vi "CMD_RETURN.vi"(6 "Gantry in":refnum<class "Gantry.lvclass">, 8 "error in (no error)":errorcluster, 10 "Arguments":string[](array[string]), 11 "gScript Interpreter in":refnum<class "gScript Interpreter.lvclass">) -> (0 "error out":errorcluster, 3 "gScript Interpreter out":refnum<class "gScript Interpreter.lvclass">, 4 "Gantry out":refnum<class "Gantry.lvclass">)   [LabVIEW 2024, in "gScript Interpreter.lvclass"]
uses:
  gScript Interpreter.lvclass
  Shared Components/Gantry Class/Gantry.lvclass
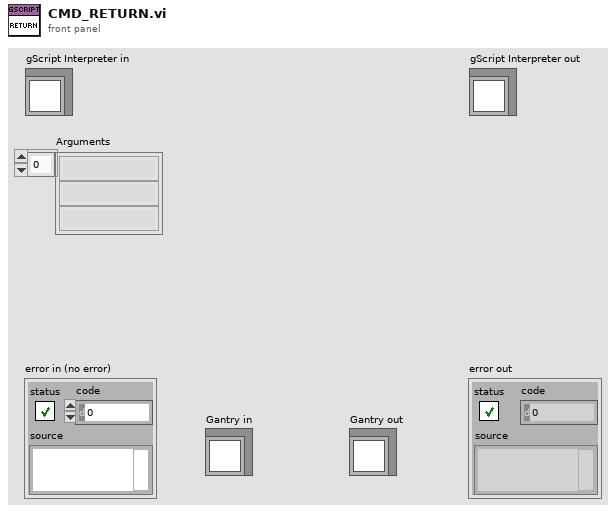
[diagram p1: front panel]
types:
  T1 = typedef "Memory Cell.ctl" = cluster{"type":T2, "x":dbl, "y":dbl, "z":dbl, "w":dbl}
  T2 = typedef "Memory Cell Type Enum.ctl" = enum16{"integer", "float", "vector", "rotation"}
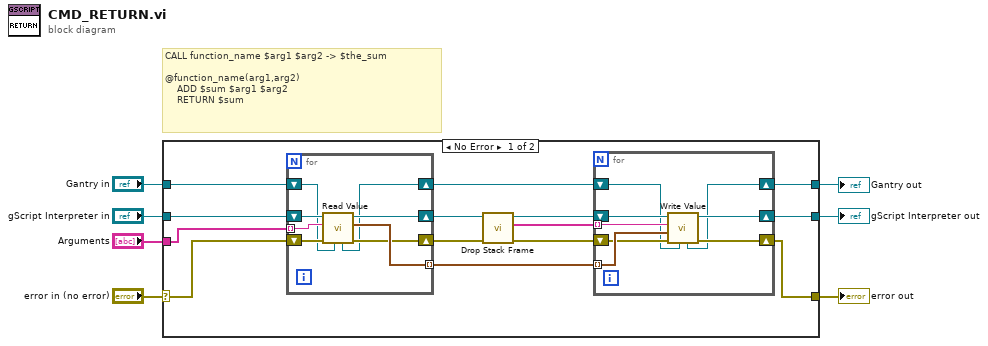
[diagram p0: block diagram]
diagram:
  # "CALL function_name $arg1 $arg2 -> $the_sum\n\n@function_name(arg1,arg2)\n    ADD $sum $arg1 $arg2\n    RETURN $sum"
  n1 = case shown="No Error" "error in (no error)" {
    selector: "error in (no error)" -> [w18 w40]
    tunnel: [w11 w40] -> w6
    tunnel: [w12 w39] -> w4
    tunnel: "gScript Interpreter in" -> [w21 w39]
    tunnel: "Arguments" -> [w20 _]
    tunnel: "Gantry in" -> [w10 w38]
    tunnel: [w8 w38] -> w1
    frame No Error {
      n2 = for {
        tunnel: w20 -> [w36] mode=indexing
        tunnel: [w35] -> w13 mode=indexing
        shift-right: [w34] -> w19
        shift-left: w21 -> [w37]
        shift-right: [w32] -> w17
        shift-left: w18 -> [w33]
        shift-right: [w30] -> w9
        shift-left: w10 -> [w31]
        n3 = call-dynamic "Read Value.vi"("Gantry in"=w31, "error in (no error)"=w33, "String in"=w36, "gScript Interpreter in"=w37) -> ("error out"=w32:errorcluster, "Memory Cell"=w35:T1, "gScript Interpreter out"=w34:refnum<class "gScript Interpreter.lvclass">, "Gantry out"=w30:refnum<class "Gantry.lvclass">)  [unwired: 4 in]
      }
      n4 = call "Drop Stack Frame.vi"("error in (no error)"=w17, "gScript Interpreter in"=w19) -> ("error out"=w15:errorcluster, "Return Bindings"=w14:string[], "gScript Interpreter out"=w16:refnum<class "gScript Interpreter.lvclass">)  [unwired: 7 in]
      n5 = for {
        tunnel: w14 -> [w27] mode=indexing
        tunnel: w13 -> [w26] mode=indexing
        shift-right: [w24] -> w11
        shift-left: w15 -> [w25]
        shift-right: [w28] -> w12
        shift-left: w16 -> [w29]
        shift-right: [w22] -> w8
        shift-left: w9 -> [w23]
        n6 = call-dynamic "Write Value.vi"("Gantry in"=w23, "error in (no error)"=w25, "Value"=w26, "Address"=w27, "gScript Interpreter in"=w29) -> ("error out"=w24:errorcluster, "gScript Interpreter out"=w28:refnum<class "gScript Interpreter.lvclass">, "Gantry out"=w22:refnum<class "Gantry.lvclass">)  [unwired: 4 in]
      }
    }
    frame Error {
    }
  }
  "error out" <- w6
  "gScript Interpreter out" <- w4
  "Gantry out" <- w1
